vi "rwFile - ConvertCoords.vi"() -> ()   [LabVIEW 2016]
uses:
  <vilib>/Utility/file.llb/Write Delimited Spreadsheet (DBL).vi
  <vilib>/Utility/file.llb/Read Delimited Spreadsheet (DBL).vi
  <vilib>/regexp/Match Regular Expression.xnode
panel:
  out "Array (stage frame, mm)":dbl[][](array[numeric])
  in  "Pixel resolution":dbl format="%#_13g"
  in  "Original Units":T1(ring)
  in  "Image Origin in XYZ Stage Coords [mm]":dbl[](array[numeric])=[38.5, -88.5, 0.0]
  in  "Source array file":path=path "E:/XYZstage+Camera_CollectedImages/12-22-2016/diagnosticSheetCoords.csv"
  in  "Clone?":bool
  in  "delimiter (\\t)":string=","
  in  "Z Array":dbl[](array[numeric])=[0.0, 0.0, 0.0, 0.0, 0.0, 0.0, 0.0, 0.0, 0.0, 0.0, 0.0, 0.0, 0.0, 0.0, 0.0, 0.0, 0.0, 0.0, 0.0, 0.0, 0.0, 0.0, 0.0, 0.0, 0.0, 0.0]
  in  "Y Array":dbl[](array[numeric])=[-32.0, -32.0, -32.0, -32.0, -32.0, -32.0, -32.0, -32.0, -32.0, -32.0, -32.0, -32.0, -32.0, -132.0, -132.0, -132.0, -132.0, -132.0, -132.0, -132.0, -132.0, -132.0, -132.0, -132.0, -132.0, -132.0]
  in  "X Array":dbl[](array[numeric])=[-709.0, -611.0, -513.0, -415.0, -317.0, -219.0, -121.0, -23.0, 75.0, 173.0, 271.0, 369.0, 467.0, 467.0, 369.0, 271.0, 173.0, 75.0, -23.0, -121.0, -219.0, -317.0, -415.0, -513.0, -611.0, -709.0]
  out "all rows":dbl[][](array[numeric])=[[-709.0, -32.0, 0.0], [-611.0, -32.0, 0.0], [-513.0, -32.0, 0.0], [-415.0, -32.0, 0.0], [-317.0, -32.0, 0.0], [-219.0, -32.0, 0.0], [-121.0, -32.0, 0.0], [-23.0, -32.0, 0.0], [75.0, -32.0, 0.0], [173.0, -32.0, 0.0], [271.0, -32.0, 0.0], [369.0, -32.0, 0.0], [467.0, -32.0, 0.0], [467.0, -132.0, 0.0], [369.0, -132.0, 0.0], [271.0, -132.0, 0.0], [173.0, -132.0, 0.0], [75.0, -132.0, 0.0], [-23.0, -132.0, 0.0], [-121.0, -132.0, 0.0], [-219.0, -132.0, 0.0], [-317.0, -132.0, 0.0], [-415.0, -132.0, 0.0], [-513.0, -132.0, 0.0], [-611.0, -132.0, 0.0], [-709.0, -132.0, 0.0]]
  in  "transpose? (no:F)":bool
  in  "Export file path (dialog if empty)":path=path "E:/XYZstage+Camera_CollectedImages/12-22-2016/diagnosticSheetCoords-transformed.csv"
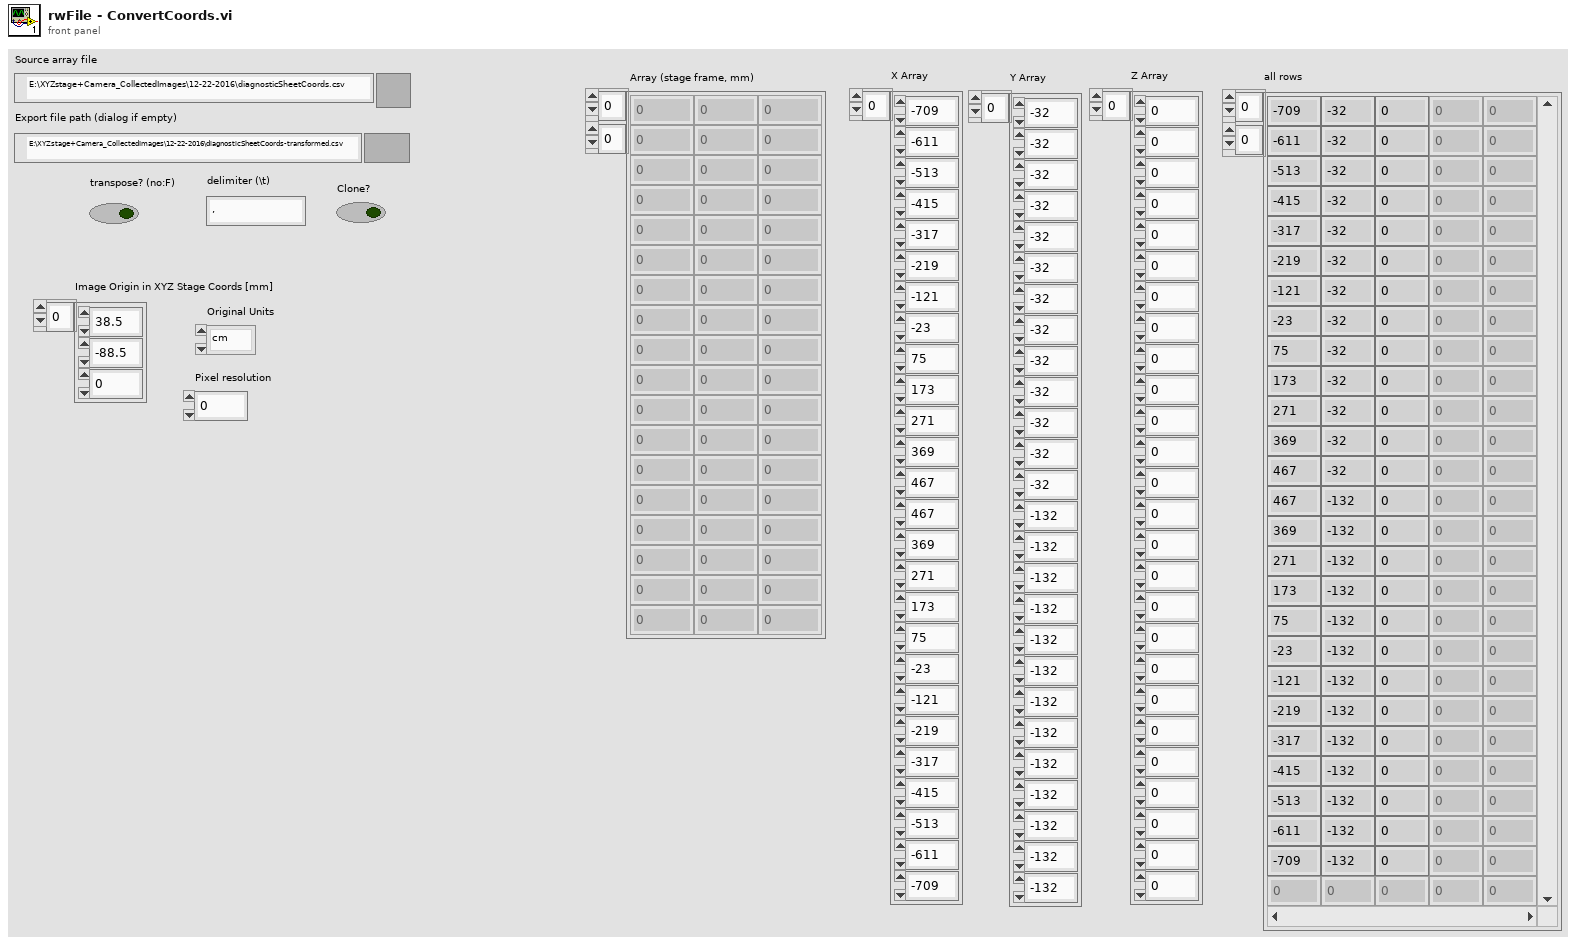
[diagram p1: front panel]
types:
  T1 = enum16{"cm", "mm", "pixels [mm/pix]", "pixels [um/pix]"}
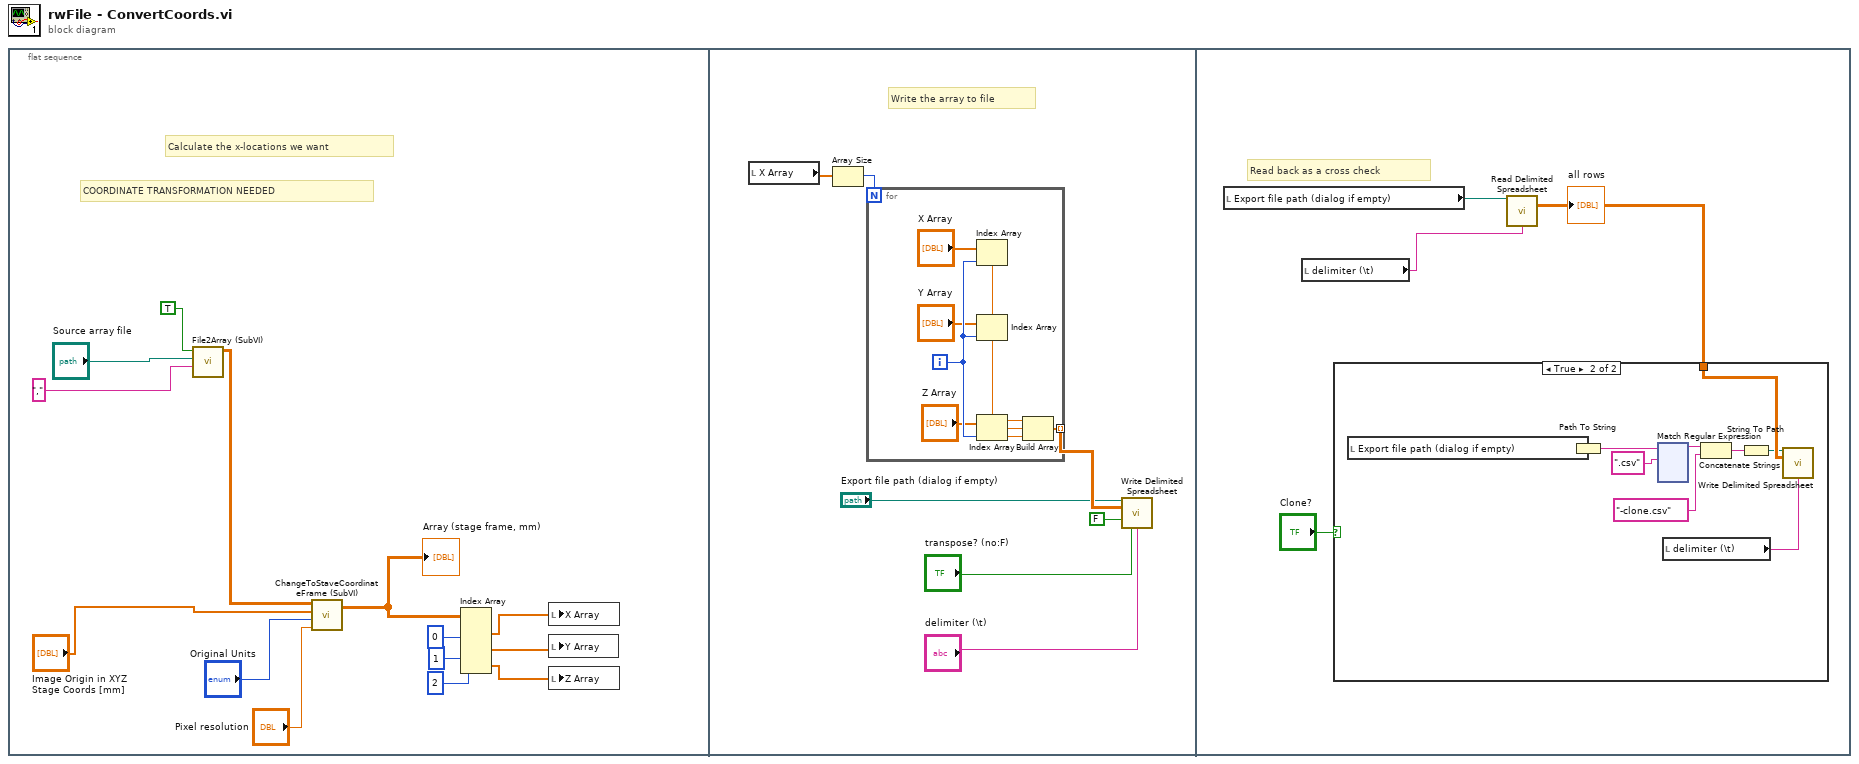
[diagram p0: block diagram]
diagram:
  n1 = flat-sequence {
    frame #0 {
      # "COORDINATE TRANSFORMATION NEEDED"
      # "Calculate the x-locations we want"
      n2 = call "File2Array (SubVI).vi"("File delimiter"=",", "Source array file"="Source array file", "Load array from file?"=TRUE) -> ("Loaded array"=w11:dbl[][])  [unwired: 7 in, 1 out]
      n3 = call "ChangeToStaveCoordinateFrame (SubVI).vi"("Loaded array (image frame)"=w11, "Image Origin in XYZ Stage Coords [mm]"="Image Origin in XYZ Stage Coords [mm]", "Units"="Original Units", "Pixel resolution"="Pixel resolution") -> ("Array (stage frame, mm)"=w7:dbl[][])  [unwired: 2 in]
      "Array (stage frame, mm)" <- w7
      n4 = Index Array(array=w7, index (col) #1=0 ("disabled index (col)"), index (col) #2=1 ("index (col)"), index (col) #3=2 ("index (col)")) -> (element #1=w3:dbl[], element #2=w2:dbl[], element #3=w1:dbl[])  [unwired: 3 in]
      n5 = local write "X Array"(w3) -> ()
      n6 = local write "Y Array"(w2) -> ()
      n7 = local write "Z Array"(w1) -> ()
    }
    frame #1 {
      # "Write the array to file"
      n8 = local read "X Array"() -> (w19:dbl[])
      n9 = Array Size(array=w19) -> (size(s)=w18:i32)
      n10 = for {
        N: w18 -> [_]
        tunnel: [w22] -> w20 mode=indexing
        i -> [w29]
        n11 = Index Array(array="X Array", index=w29) -> (element=w23:dbl)
        n12 = Index Array(array="Y Array", index=w29) -> (element=w25:dbl)
        n13 = Index Array(array="Z Array", index=w29) -> (element=w24:dbl)
        n14 = Build Array(w23, w25, w24) -> (w22:dbl[])
      }
      n15 = call-poly <vilib>:"Write Delimited Spreadsheet.vi"("file path (dialog if empty)"="Export file path (dialog if empty)", "2D data"=w20, "append to file? (new file:F)"=FALSE, "transpose? (no:F)"="transpose? (no:F)", "delimiter (\\t)"="delimiter (\\t)") -> ()  [unwired: 9 in, 2 out]
    }
    frame #2 {
      # "Read back as a cross check"
      n16 = local read "Export file path (dialog if empty)"() -> (w33:path)
      n17 = local read "delimiter (\\t)"() -> (w30:string)
      n18 = call-poly <vilib>:"Read Delimited Spreadsheet.vi"("file path (dialog if empty)"=w33, "delimiter (\\t)"=w30) -> ("all rows"=w32:dbl[][])  [unwired: 8 in, 5 out]
      "all rows" <- w32
      n19 = case shown="True" "Clone?" {
        tunnel: w32 -> [_ w42]
        frame False {
        }
        frame True {
          n20 = local read "Export file path (dialog if empty)"() -> (w41:path)
          n21 = Path To String(path=w41) -> (string=w40:string)
          n22 = xnode "Match Regular Expression"("input string"=w40, "regular expression"=".csv") -> ("before match"=w37:string)  [unwired: 4 in, 4 out]
          n23 = local read "delimiter (\\t)"() -> (w34:string)
          n24 = Concatenate Strings(w37, "-clone.csv" ("name or relative path")) -> (w36:string)
          n25 = String To Path(string=w36) -> (path=w35:path)
          n26 = call-poly <vilib>:"Write Delimited Spreadsheet.vi"("file path (dialog if empty)"=w35, "2D data"=w42, "delimiter (\\t)"=w34) -> ()  [unwired: 11 in, 2 out]
        }
      }
    }
  }
